vi "SV UFF58 Write ASCII Function (Time Waveform) (1 Ch).vi"(0 "file refnum":refnum<file>, 1 "ID lines (1-3)":T3, 2 "data precision (DBL:1)":T4=1 items=["single-precision", "double-precision"], 5 "waveform":waveform(dbl)={"t0"=timestamp(0 s since 1904-01-01), "dt"=0.0, "Y"=[]}, 11 "error in (no error)":errorcluster, 12 "DOF Identification":T2 {"response direction" items=["-Z Rotation"=-6, "-Y Rotation"=-5, "-X Rotation"=-4, "-Z Translation"=-3, "-Y Translation"=-2, "-X Translation"=-1, "Scalar"=0, "+X Translation"=1, "+Y Translation"=2, "+Z Translation"=3, "+X Rotation"=4, "+Y Rotation"=5, "+Z Rotation"=6]}) -> (4 "dup file refnum":refnum<file>, 15 "error out":errorcluster)   [LabVIEW 2017, in "SoundVib_UFF58.lvlib"]
doc: "Writes data to the UFF58 (universal file format) file specified by the <B>file refnum</B> input. This VI also writes the fields in records 1, 2, and 3, <B>ID lines (1-3)</B>. You can write a single time domain waveform, a single real frequency spectrum, or a complex frequency spectrum to a UFF file. If a frequency spectrum is in decibels, this VI converts the spectrum to linear before writing to the UFF58 file. The default instance, SV UFF58 Write ASCII Function (Time Waveform), writes a single time domain waveform to the file specified by the <B>file refnum</B> input. Wire data to the <B>file refnum</B> input to determine the polymorphic instance to use or manually select the instance."
uses:
  <vilib>/addons/Sound and Vibration/svt_UFF58/SoundVib_UFF58.lvlib
  <vilib>/addons/Sound and Vibration/svt_UFF58/subVIs/sv_UFF58 Data Precision.ctl
  <vilib>/addons/Sound and Vibration/svt_UFF58/subVIs/sv_IDLines123.ctl
  <vilib>/addons/Sound and Vibration/svt_UFF58/subVIs/sv_UFF58 Response Direction.ctl
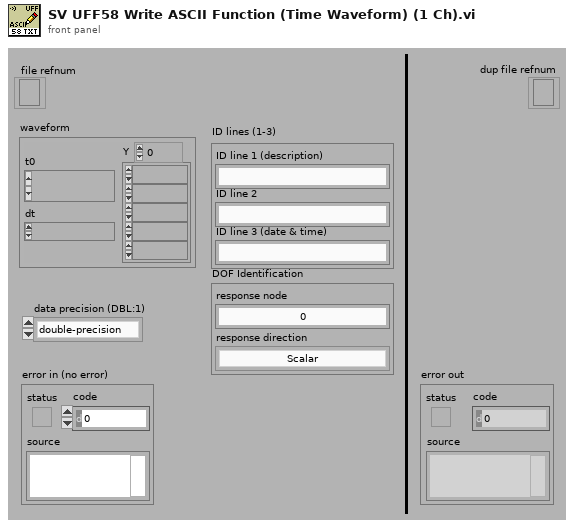
[diagram p1: front panel]
types:
  T1 = typedef "SoundVib_UFF58.lvlib/sv_UFF58 Response Direction.ctl" = i32
  T2 = cluster{"response node":i32, "response direction":T1}
  T3 = typedef "SoundVib_UFF58.lvlib/sv_IDLines123.ctl" = cluster{"ID line 1 (description)":string, "ID line 2":string, "ID line 3 (date & time)":string}
  T4 = typedef "SoundVib_UFF58.lvlib/sv_UFF58 Data Precision.ctl" = u32
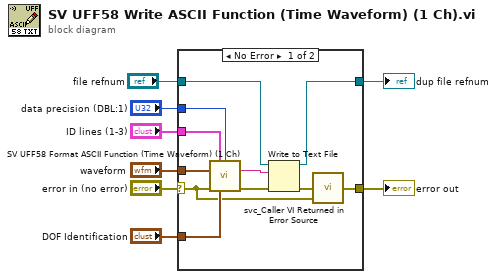
[diagram p0: block diagram]
diagram:
  n1 = case shown="No Error" "error in (no error)" {
    selector: "error in (no error)" -> [w11 w21]
    tunnel: "data precision (DBL:1)" -> [w13 _]
    tunnel: "waveform" -> [w15 _]
    tunnel: "ID lines (1-3)" -> [w17 _]
    tunnel: "DOF Identification" -> [w16 _]
    tunnel: [w9 w21] -> w3
    tunnel: "file refnum" -> [w19 w20]
    tunnel: [w18 w20] -> w1
    frame No Error {
      n2 = call <vilib>:"SV UFF58 Format ASCII Function (Time Waveform) (1 Ch).vi"("ID lines (1-3)"=w17, "data precision (DBL:1)"=w13, "waveform"=w15, "error in (no error)"=w11, "DOF Identification"=w16) -> ("UFF58 ASCII function string"=w12:string, "error out"=w14:errorcluster)  [unwired: 9 in]
      n3 = Write to Text File(file (use dialog)=w19, text=w12, error in=w14) -> (refnum out=w18:refnum<file>, error out=w10:errorcluster)  [unwired: 1 in, 1 out]
      n4 = call <vilib>:"svc_Caller VI Returned in Error Source.vi"("warning input to caller"=w11, "error in (no error)"=w10) -> ("error out"=w9:errorcluster)  [unwired: 3 in]
    }
    frame Error {
    }
  }
  "error out" <- w3
  "dup file refnum" <- w1
